vi "Ejercicio 2Feb.vi"() -> ()   [LabVIEW 2013]
panel:
  out "POTENCIA":dbl
  out "EXPONENTE":dbl
  out "BASE":dbl
  # "Generar la base y el exponente con numeros de 1-10 luego generar potencia usando \nel ciclo for"
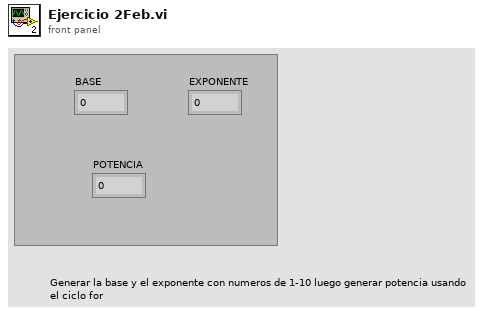
[diagram p1: front panel]
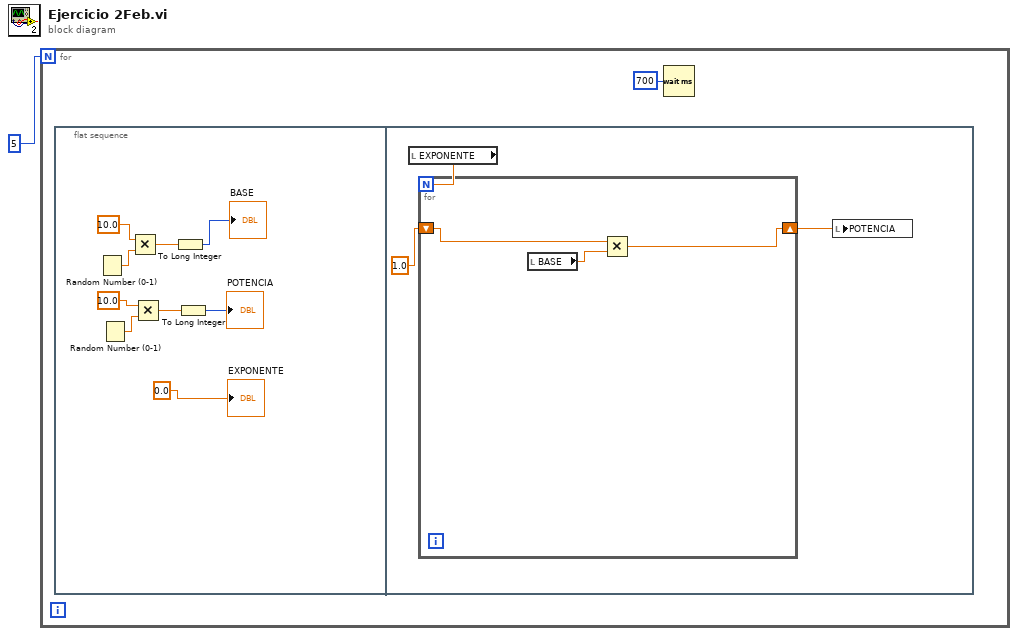
[diagram p0: block diagram]
diagram:
  n1 = for {
    N: 5 -> [_]
    n2 = flat-sequence {
      frame #0 {
        n3 = Random Number (0-1)() -> (number: 0 to 1=w11:dbl)
        n4 = Random Number (0-1)() -> (number: 0 to 1=w6:dbl)
        n5 = Multiply(x=10.0, y=w11) -> (x*y=w10:dbl)
        n6 = Multiply(x=10.0, y=w6) -> (x*y=w7:dbl)
        n7 = To Long Integer(number=w10) -> (32bit integer=→"BASE":i32)
        n8 = To Long Integer(number=w7) -> (32bit integer=→"POTENCIA":i32)
        "EXPONENTE" <- 0.0
      }
      frame #1 {
        n9 = local read "EXPONENTE"() -> (w14:dbl)
        n10 = for {
          N: w14 -> [_]
          shift-right: [w15] -> w12
          shift-left: 1.0 -> [w17]
          n11 = local read "BASE"() -> (w16:dbl)
          n12 = Multiply(x=w17, y=w16) -> (x*y=w15:dbl)
        }
        n13 = local write "POTENCIA"(w12) -> ()
      }
    }
    n14 = Wait (ms)(milliseconds to wait=700) -> ()  [unwired: 1 out]
  }
